vi "Test Nesetd Cluster.vi"(11 "Test Case In":refnum<class "Describe Variant Test.lvclass">) -> (0 "error out":errorcluster, 3 "Test Case Out":refnum<class "Describe Variant Test.lvclass">)   [LabVIEW 2020, in "Describe Variant Test.lvclass"]
uses:
  Describe Variant Test.lvclass
  C:/Program Files (x86)/National Instruments/LabVIEW 2020/vi.lib/Astemes/LUnit/Test Case.lvclass
  <vilib>/Astemes/LUnit/Test Case.lvclass/Test Case.ctl
  7c39a56f-5538-4c7e-9d72-f297bb98ba6b.vi
  <vilib>/Astemes/LUnit/Core/LUnit Test Case/Private/Append Pass Result.vi
  <vilib>/Astemes/LUnit/Core/LUnit Test Case/Private/Append Fail Result.vi
  7c39a56f-5538-4c7e-9d72-f297bb98ba6b.vi/9c5d11cd-9439-4240-a1ee-d9baace9c924.vi
  <vilib>/Astemes/LUnit/Core/LUnit Test Case/Private/Run In UI.vi
  <vilib>/Utility/error.llb/Clear Errors.vi
  source/Framework/Utilities/Utilities.lvlib
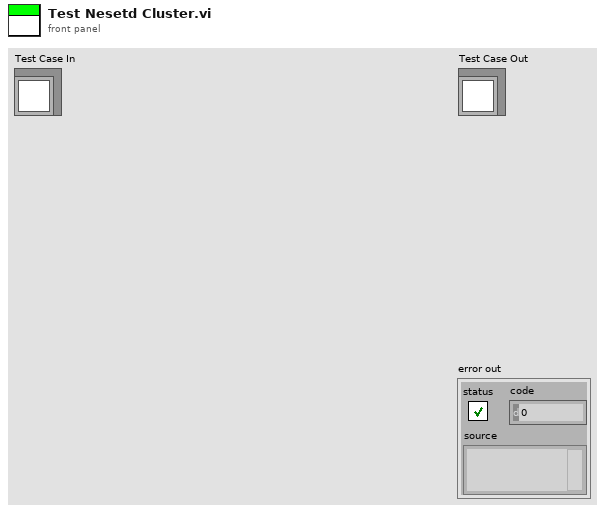
[diagram p1: front panel]
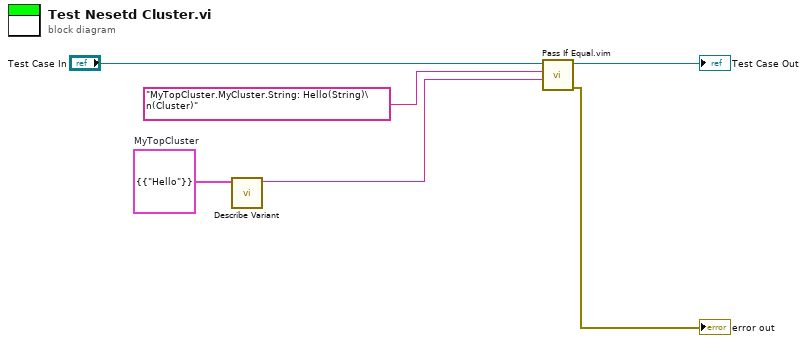
[diagram p0: block diagram]
diagram:
  w1 = cluster{"MyCluster":cluster{"String":string}} {"MyCluster"={"String"="Hello"}}  # MyTopCluster
  n1 = call "Describe Variant.vi"("Variant"=w1) -> ("Variant Description"=w2:string)  [unwired: 8 in, 2 out]
  n2 = call "Pass If Equal.vim"("Actual"=w2, "Expected"="MyTopCluster.MyCluster.String: Hello(String)\n(Cluster)", "LUnit Test Case In"="Test Case In") -> ("error out"=→"error out":errorcluster, "LUnit Test Case Out"=→"Test Case Out":refnum<class "Describe Variant Test.lvclass">)  [unwired: 7 in]
